vi "Instrument - Manual Object.vi"() -> ()   [LabVIEW 2015, in "Instrument Workspace Objects.lvlib"]
doc: "Sample numeric display item."
uses:
  Instrument Workspace Objects.lvlib
  <vilib>/NI Veristand/Display Template Support/Display Template Support.llb/cluster_Screen Item Settings.ctl
  <vilib>/NI Veristand/Display Template Support/Display Template Support.llb/cluster_Graph Scale Settings.ctl
  <vilib>/NI Veristand/Display Template Support/Display Template Support.llb/cluster_Graph Plot Settings.ctl
  Shared/Types/Response Wait Type.ctl
  NationalInstruments.VeriStand.SystemStorage
  <vilib>/NI Veristand/Display Template Support/Display Template Support.llb/enum_Display Template Handler Minimal To Widget Msg.ctl
  <vilib>/NI Veristand/Display Template Support/Display Template Support.llb/enum_Display Template Handler Minimal To Workspace.ctl
  Types/State Variables.ctl
  <vilib>/NI Veristand/Execution/Workspace/WorkspaceAPI.ctl
  <userlib>/STM/TCP/stm_TCP Connection Info.ctl
  <userlib>/STM/_SubVIs/stm_MetaDataElement.ctl
  Types/CD Saved State.ctl
  <vilib>/NI Veristand/Execution/Workspace/SystemStateEventRef.ctl
  <vilib>/NI Veristand/Execution/Workspace/Target State Info.ctl
  <vilib>/NI Veristand/Execution/Workspace/Target State.ctl
  <vilib>/NI Veristand/Execution/Workspace/SystemStateRegEventRef.ctl
  Engine/Types/Buffered RT Instrument Command.ctl
  <vilib>/NI Veristand/Display Template Support/Display Template Support.llb/sub_Display Template Handler Custom.vi
  Host API/Instrument CD Host API.lvlib
  Shared/Instrument Addon Shared.lvlib
  Engine/Instrument Addon Engine.lvlib
  <vilib>/NI Veristand/Execution/Workspace/NI_VS Workspace ExecutionAPI.lvlib
  NationalInstruments.VeriStand.ClientAPI
panel:
  in  "NIVS.Gateway IP Address":string
  out "Device":string
  in  "NIVS.System Definition Root":refnum<k24>
  out "Error Report":errorcluster
  in  "Response?":bool
  out "Timed Out?":bool
  out "Response":string
  in  "Send":bool
  in  "Wait Value":dbl=100.0 format="%#_p"
  in  "Wait Type":T1
  in  "Command":string
  in  "Item.Data":T2
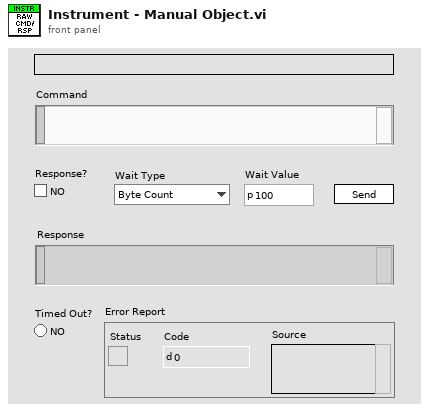
[diagram p1: front panel]
types:
  T1 = typedef "Instrument Addon Shared.lvlib/Response Wait Type.ctl" = enum16{"Byte Count", "Wait sec"}
  T2 = typedef "cluster_Screen Item Settings.ctl" = cluster{"Template VI":string, "Position X":i32, "Position Y":i32, "Custom":string, "Show Title Bar":bool, "ID":i32, "Always On Top":bool, "Allow Resize":bool, "Allow Minimize":bool, "Allow Close":bool, "Size to Screen":bool, "Screen.ID":i32, "State":enum16{"Normal", "New"}, "Title":string, "Window Bounds":cluster{"[0]":i16, "[1]":i16, "[2]":i16, "[3]":i16}, "Channel Ref":u64, "Unit":string, "Default Units?":bool, "Flash Limit?":bool, "Color 1":u32, "Color 2":u32, "Color 3":u32, "Color 4":u32, "Bck Color":u32, "Fore Color":u32, "Limit 1":dbl, "Limit 2":dbl, "Limit 3":dbl, "Limit 4":dbl, "Limit Mode 1":i32, "Limit Mode 2":i32, "Limit Mode 3":i32, "Limit Mode 4":i32, "Scale Precision":i32, "Scale Min":dbl, "Scale Max":dbl, "Format":i32, "Precision":i32, "Background Type":i32, "IDs":i32[], "Units":string[], "Labels":string[], "Scale Factor":dbl, "Scale Offset":dbl, "YScale Index":u32[], "XScale":T3, "YScales":T3[], "Plots":T4[], "Update Period":dbl, "History Length":dbl, "My.Ref":refnum<vi>, "Is Control?":bool, "Channel Paths":string[], "Custom Data":variant}
  T3 = typedef "cluster_Graph Scale Settings.ctl" = cluster{"Format":u8, "Precision":u8, "Fit":u8, "Label":string, "Use Default Label":bool, "Label Visible":bool, "Min":dbl, "Max":dbl}
  T4 = typedef "cluster_Graph Plot Settings.ctl" = cluster{"Bar Style":u8, "Fill To":i16, "Fill/PtColor":u32, "Line Style":u8, "Line Width":u8, "Color":u32, "Interp":u8, "Point Style":u8}
  T5 = typedef "Instrument Workspace Objects.lvlib/State Variables.ctl" = cluster{"UI.Device":refnum<vi>, "NIVS.CachedDataRef":refnum<user-event>, "NIVS.LaunchRef":refnum<user-event>, "NIVS.SysDefRoot":refnum<k24>, "NIVS.Workspace":T6, "Connection.Info":T7, "NIVS.CachedData":T9, "NIVS.SystemStateRefs":T10, "NIVS.UserEventRefs":cluster{"SystemChangeEventRef":T11, "Event Registration Refnum":refnum<event-registration>}, "Workspace.Connected?":bool}
  T6 = typedef "NI_VS Workspace ExecutionAPI.lvlib/WorkspaceAPI.ctl" = refnum<k24>
  T7 = typedef "stm_TCP Connection Info.ctl" = cluster{"connection ID":refnum<k5>, "Meta data":T8[]}
  T8 = typedef "stm_MetaDataElement.ctl" = string
  T9 = typedef "Instrument Workspace Objects.lvlib/CD Saved State.ctl" = cluster{"CD Path":string, "CD IP":string}
  T10 = typedef "NI_VS Workspace ExecutionAPI.lvlib/SystemStateEventRef.ctl" = cluster{"CustDatRef":refnum<user-event>, "EvtRef":refnum<k27>, "Target State User Event":refnum<user-event>}
  T11 = typedef "NI_VS Workspace ExecutionAPI.lvlib/SystemStateRegEventRef.ctl" = refnum<event-registration>
  T12 = typedef "enum_Display Template Handler Minimal To Workspace.ctl" = cluster{"Operation":enum16{"SetCustomData", "DeleteItem"}, "Data":variant}
  T13 = typedef "enum_Display Template Handler Minimal To Widget Msg.ctl" = enum16{"Stop", "LaunchConfigDialog"}
  T14 = typedef "Instrument Addon Engine.lvlib/Buffered RT Instrument Command.ctl" = cluster{"Command":string, "Response Expected?":bool, "Wait Type":T1, "Wait Value":dbl}
  T15 = typedef "NI_VS Workspace ExecutionAPI.lvlib/SystemState.ctl" = u8
  T16 = enum8{"Enabled", "Disabled", "Disabled and Grayed Out"}
  T17 = cluster{"SystemChangeEventRef":T11, "Event Registration Refnum":refnum<event-registration>}
  T18 = typedef "Instrument Addon Engine.lvlib/Buffered RT Instrument Request.ctl" = cluster{"Response":string, "Error":errorcluster}
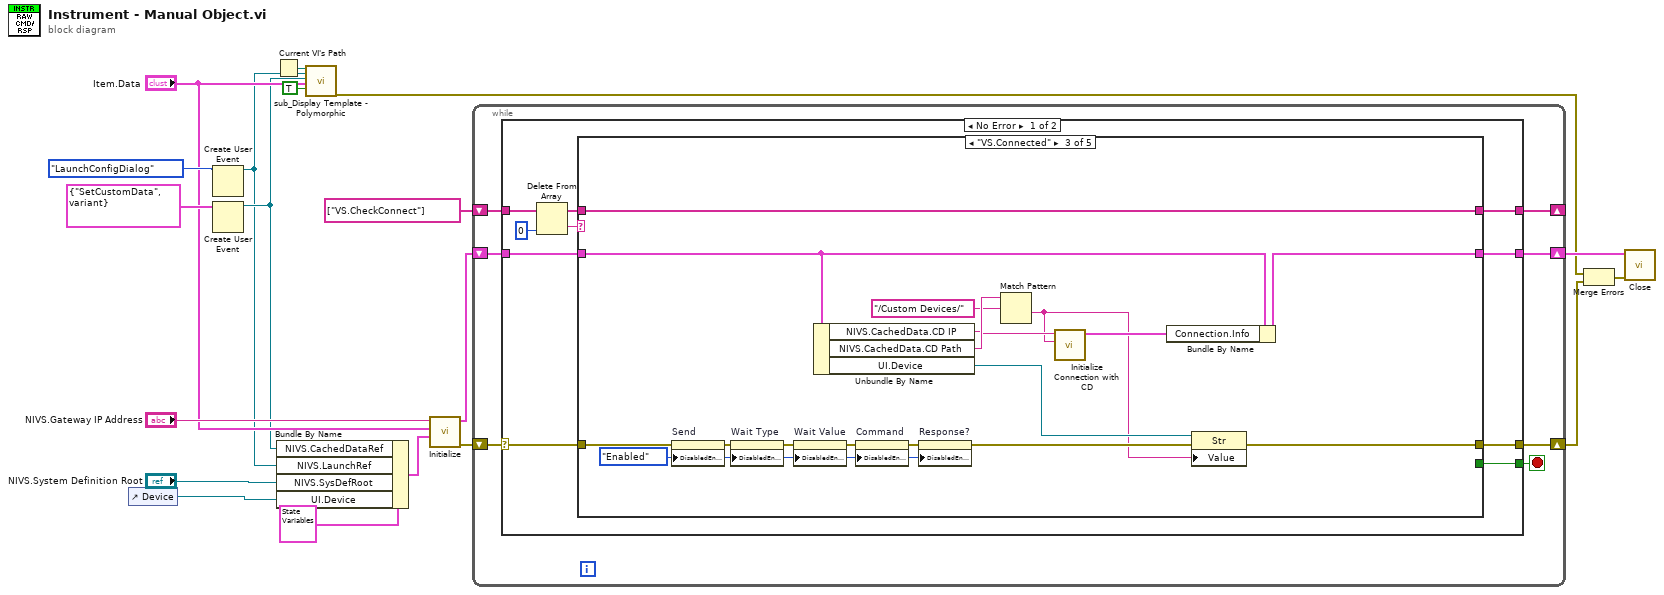
[diagram p0: block diagram]
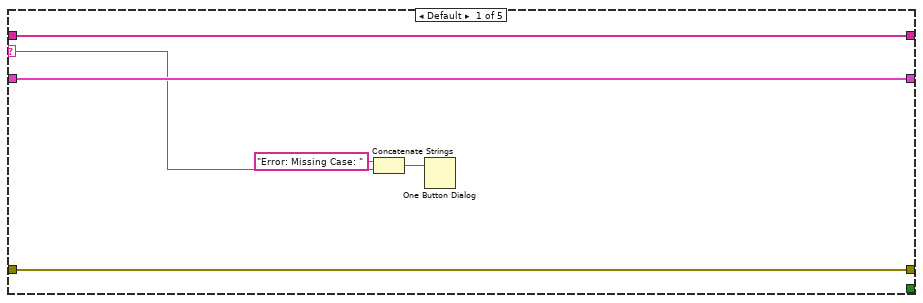
[diagram p2: hidden frame]
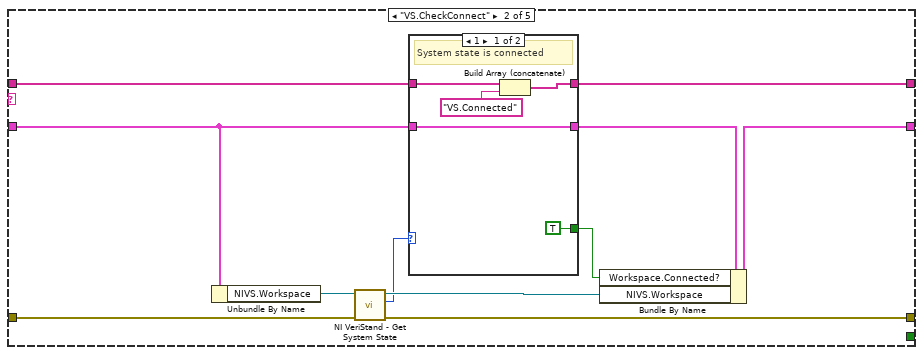
[diagram p3: hidden frame]
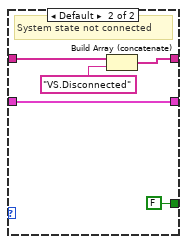
[diagram p4: hidden frame]
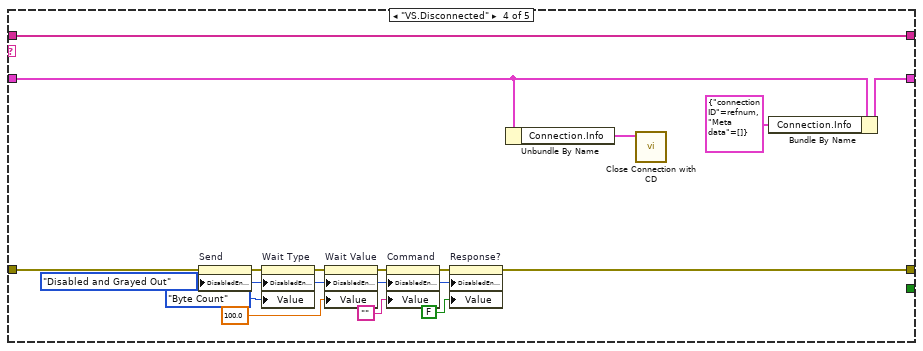
[diagram p5: hidden frame]
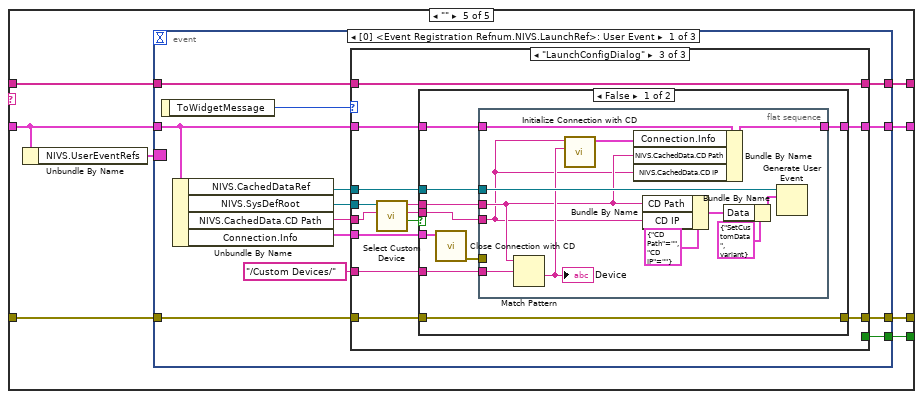
[diagram p6: hidden frame]
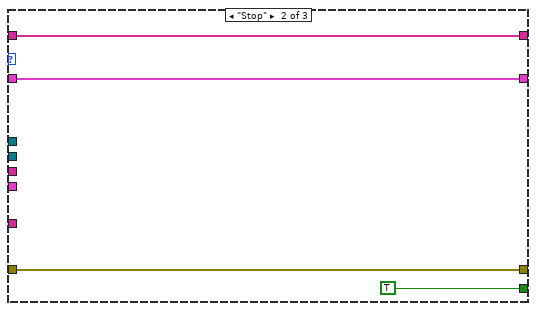
[diagram p8: hidden frame]
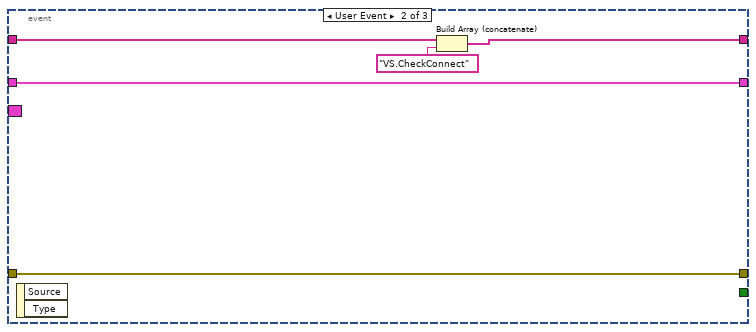
[diagram p10: hidden frame]
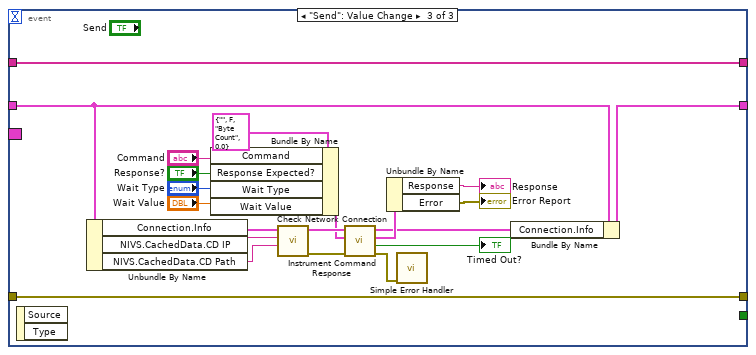
[diagram p11: hidden frame]
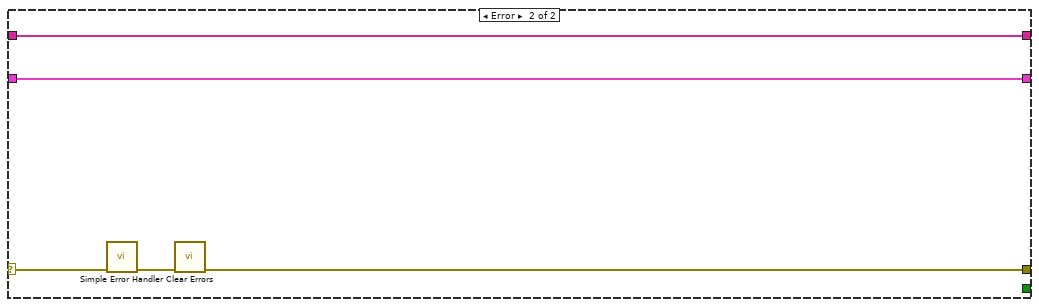
[diagram p12: hidden frame]
diagram:
  n1 = control-ref of="Device"() -> (w11:refnum<vi>)
  n2 = Create User Event(user event datatype=enum_Display_Template_Handler_Minimal_To_Widget_Msg."LaunchConfigDialog" ("ToWidgetMessage")) -> (user event=w5:refnum<user-event>)  [unwired: 1 in, 1 out]
  n3 = Create User Event(user event datatype=T12 {"Operation"=enum."SetCustomData", "Data"=variant} ("Data")) -> (user event=w6:refnum<user-event>)  [unwired: 1 in, 1 out]
  n4 = Current VI's Path() -> (path=w17:path)
  n5 = Bundle By Name(cluster=T5 {"UI.Device"=refnum, "NIVS.CachedDataRef"=refnum, "NIVS.LaunchRef"=refnum, "NIVS.SysDefRoot"=refnum, "NIVS.Workspace"=refnum, "Connection.Info"={"connection ID"=refnum, "Meta data"=[]}, "NIVS.CachedData"={"CD Path"="", "CD IP"=""}, "NIVS.SystemStateRefs"={"CustDatRef"=refnum, "EvtRef"=refnum, "Target State User Event"=refnum}, "NIVS.UserEventRefs"={"SystemChangeEventRef"=refnum, "Event Registration Refnum"=refnum}, "Workspace.Connected?"=FALSE} ("State Variables in"), "NIVS.CachedDataRef"=w6, "NIVS.LaunchRef"=w5, "NIVS.SysDefRoot"="NIVS.System Definition Root", "UI.Device"=w11) -> (w9:T5)
  n6 = call-poly <vilib>:"sub_Display Template - Polymorphic.vi"("Parent.Path"=w17, "ToWidgetEvent"=w5, "ToWorkspace"=w6, "Item.Data"="Item.Data", "Resizable"=TRUE) -> ("error out"=w3:errorcluster)  [unwired: 1 in, 13 out]
  n7 = call "Initialize.vi"("State Variables in"=w9, "Item.Data"="Item.Data", "NIVS.Gateway IP Address"="NIVS.Gateway IP Address") -> ("error out"=w14:errorcluster, "State Variables out"=w8:T5)  [unwired: 7 in]
  n8 = while {
    shift-right: [w25] -> w4
    shift-left: w14 -> [w22]
    shift-right: [w23] -> w7
    shift-left: w8 -> [w24]
    shift-right: [w20] -> _
    shift-left: string[] ["VS.CheckConnect"] -> [w21]
    stop <- w26 stop-if-true
    n9 = case shown="No Error" w22 {
      selector: w22 -> [w32 w188]
      tunnel: [w36 _] -> w26
      tunnel: [w35 w187] -> w25
      tunnel: w24 -> [w34 w191]
      tunnel: [w33 w191] -> w23
      tunnel: w21 -> [w30 w190]
      tunnel: [w27 w190] -> w20
      frame No Error {
        n10 = Delete From Array(array=w30, index=0) -> (deleted portion=w29:string, array with subset deleted=w28:string[])  [unwired: 1 in]
        n11 = case shown="\"VS.Connected\"" w29 {
          selector: w29 -> [w39 _ _ _ _]
          tunnel: [_ _ _ _ w104] -> w36
          tunnel: [w41 w46 w75 w85 w103] -> w35
          tunnel: w34 -> [w42 w48 w72 w93 w101]
          tunnel: [w42 w45 w71 w92 w100] -> w33
          tunnel: w32 -> [w41 w47 w80 w96 w99]
          tunnel: w28 -> [w40 w44 w79 w95 w97]
          tunnel: [w40 w43 w79 w95 w98] -> w27
          frame Default {
            n12 = Concatenate Strings("Error: Missing Case: " ("string"), w39) -> (w38:string)
            n13 = One Button Dialog(message=w38) -> ()  [unwired: 1 in, 1 out]
          }
          frame "VS.CheckConnect" {
            n14 = Unbundle By Name(w48) -> ("NIVS.Workspace"=w52:T6)
            n15 = call <vilib>:"NI VeriStand - Get System State.vi"("error in (no error)"=w47, "WorkspaceManager in"=w52) -> ("error out"=w46:errorcluster, "System State"=w49:T15, "WorkspaceManager  out"=w53:T6)  [unwired: 5 in, 2 out]
            n16 = case shown="1" w49 {
              tunnel: [w58 w63] -> w43
              tunnel: [w56 w61] -> w50
              tunnel: w48 -> [w56 w61]
              tunnel: [TRUE FALSE] -> w51
              tunnel: w44 -> [w54 w59]
              frame 1 {
                # "System state is connected"
                n17 = Build Array (concatenate)(w54, "VS.Connected") -> (w58:string[])
              }
              frame Default {
                # "System state not connected"
                n18 = Build Array (concatenate)(w59, "VS.Disconnected") -> (w63:string[])
              }
            }
            n19 = Bundle By Name(cluster=w50, "Workspace.Connected?"=w51, "NIVS.Workspace"=w53) -> (w45:T5)
          }
          frame "VS.Connected" {
            w65 = T16."Enabled" ("Disabled")
            n20 = property on="Send" class="Bool"(error in=w80, "DisabledEnum"=w65) -> (error out=w67:errorcluster)  [unwired: 1 in, 1 out]
            n21 = property on="Wait Type" class="Enum (strict)"(error in=w67, "DisabledEnum"=w65) -> (error out=w70:errorcluster)  [unwired: 1 in, 1 out]
            n22 = property on="Wait Value" class="DigNum (strict)"(error in=w70, "DisabledEnum"=w65) -> (error out=w69:errorcluster)  [unwired: 1 in, 1 out]
            n23 = Unbundle By Name(w72) -> ("NIVS.CachedData.CD IP"=w77:string, "NIVS.CachedData.CD Path"=w78:string, "UI.Device"=w74:refnum<vi>)
            n24 = property on="Command" class="Str"(error in=w69, "DisabledEnum"=w65) -> (error out=w68:errorcluster)  [unwired: 1 in, 1 out]
            n25 = property on="Response?" class="Bool (strict)"(error in=w68, "DisabledEnum"=w65) -> (error out=w66:errorcluster)  [unwired: 1 in, 1 out]
            n26 = Match Pattern(string=w78, regular expression="/Custom Devices/") -> (after substring=w64:string)  [unwired: 1 in, 3 out]
            n27 = call "Initialize Connection with CD.vi"("TCP Service"=w64, "IP Address"=w77) -> ("Connection Info Out"=w73:T7)  [unwired: 8 in, 1 out]
            n28 = Bundle By Name(cluster=w72, "Connection.Info"=w73) -> (w71:T5)
            n29 = property class="Str"(reference=w74, error in=w66, "Value"=w64) -> (error out=w75:errorcluster)  [unwired: 1 out]
          }
          frame "VS.Disconnected" {
            w86 = T16."Disabled and Grayed Out" ("Disabled")
            n30 = property on="Send" class="Bool"(error in=w96, "DisabledEnum"=w86) -> (error out=w87:errorcluster)  [unwired: 1 in, 1 out]
            n31 = property on="Wait Type" class="Enum (strict)"(error in=w87, "DisabledEnum"=w86, "Value"=Response_Wait_Type."Byte Count" ("Wait Type")) -> (error out=w90:errorcluster)  [unwired: 1 in, 1 out]
            n32 = property on="Wait Value" class="DigNum (strict)"(error in=w90, "DisabledEnum"=w86, "Value"=100.0 ("Wait Value")) -> (error out=w89:errorcluster)  [unwired: 1 in, 1 out]
            n33 = property on="Command" class="Str"(error in=w89, "DisabledEnum"=w86, "Value"="") -> (error out=w88:errorcluster)  [unwired: 1 in, 1 out]
            n34 = property on="Response?" class="Bool (strict)"(error in=w88, "DisabledEnum"=w86, "Value"=FALSE ("Response?")) -> (error out=w85:errorcluster)  [unwired: 1 in, 1 out]
            n35 = Unbundle By Name(w93) -> ("Connection.Info"=w94:T7)
            n36 = call "Close Connection with CD.vi"("Connection Info Out"=w94) -> ()  [unwired: 10 in, 1 out]
            n37 = Bundle By Name(cluster=w93, "Connection.Info"=T7 {"connection ID"=refnum, "Meta data"=[]}) -> (w92:T5)
          }
          frame "" {
            n38 = Unbundle By Name(w101) -> ("NIVS.UserEventRefs"=w102:T17)
            n39 = event shown="[0] <Event Registration Refnum.NIVS.LaunchRef>: User Event" {
              selector: w102 -> [_ _ _]
              dyn-events: _ -> [_ _ _]
              timeout: _ -> [_ _ _]
              tunnel: [w116 _ _] -> w104
              tunnel: [w115 w162 w168] -> w100
              tunnel: w99 -> [w107 w161 w167]
              tunnel: [w108 w161 w167] -> w103
              tunnel: w101 -> [w113 w162 w169]
              tunnel: [w106 w163 w166] -> w98
              tunnel: w97 -> [w105 w164 w166]
              event User Event {
                n40 = event-data() -> ("ToWidgetMessage"=w117:T13)  [unwired: 1 out]
                n41 = Unbundle By Name(w113) -> ("NIVS.CachedDataRef"=w114:refnum<user-event>, "NIVS.SysDefRoot"=w112:refnum<k24>, "NIVS.CachedData.CD Path"=w111:string, "Connection.Info"=w110:T7)
                n42 = case shown="\"LaunchConfigDialog\"" w117 {
                  tunnel: [_ TRUE _] -> w116
                  tunnel: w114 -> [_ _ w137]
                  tunnel: w112 -> [_ _ w136]
                  tunnel: w110 -> [_ _ w132]
                  tunnel: [w120 w123 w131] -> w115
                  tunnel: w113 -> [w120 w123 w130]
                  tunnel: w111 -> [_ _ w129]
                  tunnel: "/Custom Devices/" ("regular expression") -> [_ _ w128]
                  tunnel: [w119 w122 w127] -> w108
                  tunnel: w107 -> [w119 w122 w126]
                  tunnel: [w118 w121 w125] -> w106
                  tunnel: w105 -> [w118 w121 w125]
                  frame Default {
                  }
                  frame "Stop" {
                  }
                  frame "LaunchConfigDialog" {
                    n43 = call "Select Custom Device.vi"("CD Path"=w129, "NIVS.System Definition Root"=w136) -> ("Cancelled?"=w135:bool, "IP Address"=w134:string, "Custom Device Path Out"=w133:string)  [unwired: 7 in]
                    n44 = case shown="False" w135 {
                      tunnel: w137 -> [w146 _]
                      tunnel: w134 -> [w143 _]
                      tunnel: w133 -> [w144 _]
                      tunnel: w128 -> [w145 _]
                      tunnel: w132 -> [w142 _]
                      tunnel: [w140 w160] -> w131
                      tunnel: w130 -> [w139 w160]
                      tunnel: [w138 w159] -> w127
                      tunnel: w126 -> [w138 w159]
                      frame False {
                        n45 = call "Close Connection with CD.vi"("Connection Info Out"=w142) -> ("error out"=w141:errorcluster)  [unwired: 10 in]
                        n46 = flat-sequence {
                          tunnel: w146 -> [w158]
                          tunnel: w145 -> [w155]
                          tunnel: w144 -> [w150]
                          tunnel: w143 -> [w149]
                          tunnel: w141 -> [_]
                          tunnel: [w152] -> w140
                          tunnel: w139 -> [w153]
                          frame #0 {
                            n47 = Match Pattern(string=w150, regular expression=w155) -> (after substring=w154:string)  [unwired: 1 in, 3 out]
                            "Device" <- w154
                            n48 = call "Initialize Connection with CD.vi"("TCP Service"=w154, "IP Address"=w149) -> ("Connection Info Out"=w148:T7)  [unwired: 8 in, 1 out]
                            n49 = Bundle By Name(cluster=w153, "Connection.Info"=w148, "NIVS.CachedData.CD Path"=w150, "NIVS.CachedData.CD IP"=w149) -> (w152:T5)
                            n50 = Bundle By Name(cluster=T9 {"CD Path"="", "CD IP"=""}, "CD Path"=w150, "CD IP"=w149) -> (w147:T9)
                            n51 = Bundle By Name(cluster=T12 {"Operation"=enum."SetCustomData", "Data"=variant} ("event data"), "Data"=w147) -> (w156:T12)
                            n52 = Generate User Event(user event=w158, event data cluster=w156) -> ()  [unwired: 2 in, 2 out]
                          }
                        }
                      }
                      frame True {
                      }
                    }
                  }
                }
              }
              event User Event {
                n53 = event-data() -> ()  [unwired: 3 out]
                n54 = Build Array (concatenate)(w164, "VS.CheckConnect") -> (w163:string[])
              }
              event "Send": Value Change {
                n55 = event-data() -> ()  [unwired: 3 out]
                n56 = Unbundle By Name(w169) -> ("Connection.Info"=w171:T7, "NIVS.CachedData.CD IP"=w186:string, "NIVS.CachedData.CD Path"=w185:string)
                n57 = Bundle By Name(cluster=T14 {"Command"="", "Response Expected?"=FALSE, "Wait Type"=enum."Byte Count", "Wait Value"=0.0} ("Command Parameters"), "Command"="Command", "Response Expected?"="Response?", "Wait Type"="Wait Type", "Wait Value"="Wait Value") -> (w178:T14)
                n58 = call "Check Network Connection.vi"("CD Path"=w185, "IP Address"=w186, "Connection Info"=w171) -> ("error out"=w183:errorcluster, "Connection Info Out"=w184:T7)  [unwired: 7 in]
                n59 = call "Instrument Command Response.vi"("error in (no error)"=w183, "Command Parameters"=w178, "Connection Info"=w184) -> ("error out"=w173:errorcluster, "Timed Out?"=→"Timed Out?":bool, "Response"=w176:T18, "Connection Info Out"=w170:T7)  [unwired: 5 in]
                n60 = Unbundle By Name(w176) -> ("Response"=→"Response":string, "Error"=→"Error Report":errorcluster)
                n61 = call <vilib>:"Simple Error Handler.vi"("error in (no error)"=w173) -> ()  [unwired: 4 in, 5 out]
                n62 = Bundle By Name(cluster=w169, "Connection.Info"=w170) -> (w168:T5)
              }
            }
          }
        }
      }
      frame Error {
        n63 = call <vilib>:"Simple Error Handler.vi"("error in (no error)"=w188) -> ("error out"=w189:errorcluster)  [unwired: 4 in, 4 out]
        n64 = call <vilib>:"Clear Errors.vi"("error in (no error)"=w189) -> ("error out"=w187:errorcluster)  [unwired: 5 in, 1 out]
      }
    }
  }
  n65 = Merge Errors(w3, w4) -> (w2:errorcluster)
  n66 = call "Close.vi"("error in (no error)"=w2, "State Variables in"=w7) -> ()  [unwired: 10 in]
